vi "Test Child Class Methods.vi"() -> ()   [LabVIEW 2014]
uses:
  TypeDefs/STEP State.ctl
  Measurement/Measurement.lvclass
  STEP/STEP.lvclass
  APIs/Message Queue/Message Cluster.ctl
  AutoZero/AutoZero.lvclass
  Measurement wRelev/Measurement wRelev.lvclass
  Measurement wMaster/Measurement wMaster.lvclass
  Relev/Relev.lvclass
  Mastering/Mastering.lvclass
  Scale Calibration/Scale Calibration.lvclass
  APIs/Message Queue/WINFAS 2 Message Queue.lvlib
  SeqLoop.lvlib
panel:
  out "Array":T1(array[cluster])
  in  "Class":T2(ring)
  in  "STEP State 2":T3=enum."Advance OK"
  in  "STEP State":T3=enum."First Call"
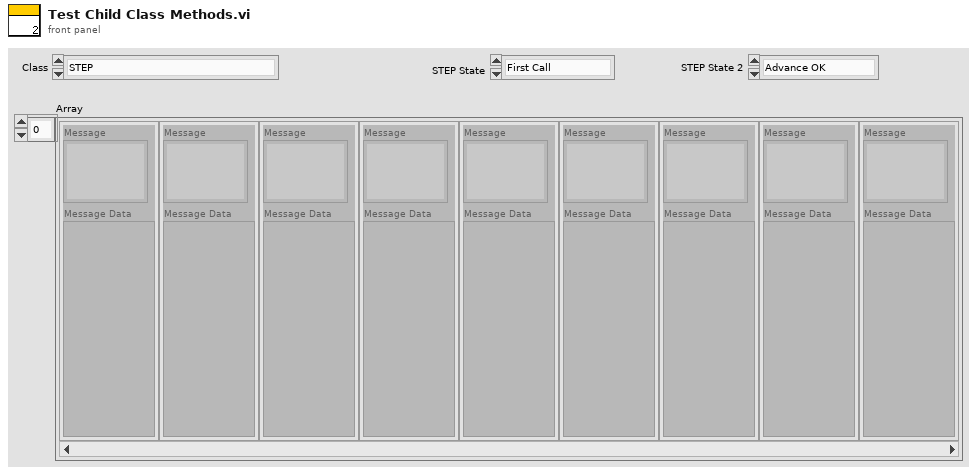
[diagram p1: front panel]
types:
  T1 = cluster{"Message":string, "Message Data":variant}[]
  T2 = enum16{"STEP", "Measurement", "AutoZero", "Measurement wRelev", "Measurement wMaster", "Relev", "Mastering", "Scale Calibration"}
  T3 = typedef "SeqLoop.lvlib/STEP State.ctl" = enum16{"Stopped", "First Call", "Idle...", "Advance OK", "Alarm", "Output Security", "Error"}
  T4 = typedef "WINFAS 2 Message Queue.lvlib/Message Cluster.ctl" = cluster{"Message":string, "Message Data":variant}
  T5 = cluster{"Message":string, "Message Data":variant}
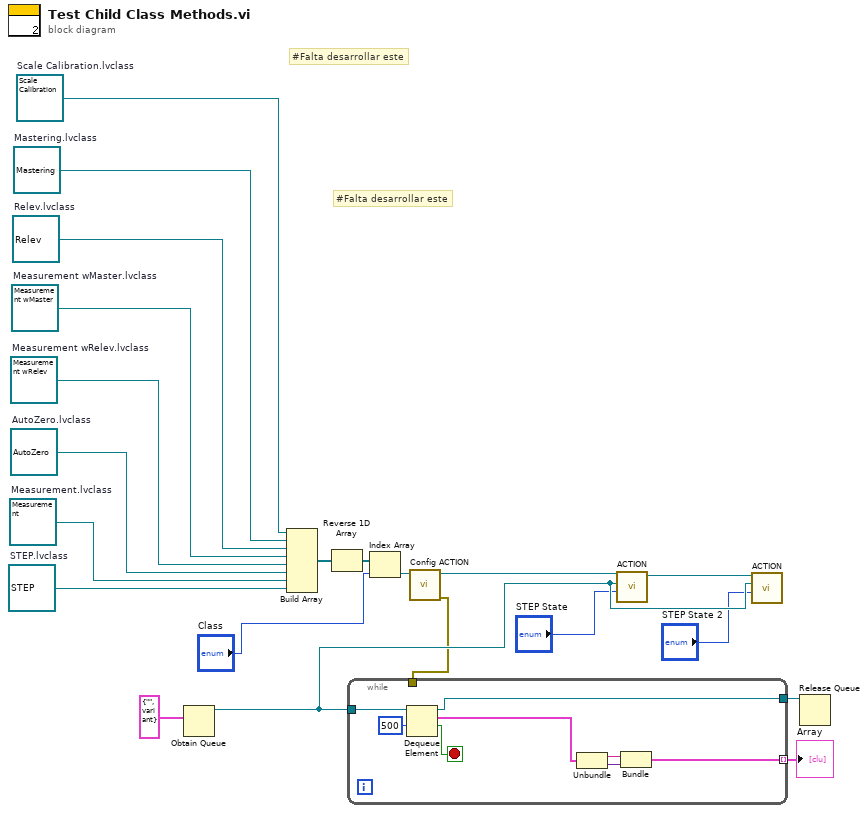
[diagram p0: block diagram]
diagram:
  w5 = refnum<class "Scale Calibration.lvclass"> refnum  # Scale Calibration.lvclass
  w6 = refnum<class "Mastering.lvclass"> refnum  # Mastering.lvclass
  w7 = refnum<class "Relev.lvclass"> refnum  # Relev.lvclass
  w8 = refnum<class "Measurement wMaster.lvclass"> refnum  # Measurement wMaster.lvclass
  w9 = refnum<class "Measurement wRelev.lvclass"> refnum  # Measurement wRelev.lvclass
  w10 = refnum<class "AutoZero.lvclass"> refnum  # AutoZero.lvclass
  w21 = refnum<class "STEP.lvclass"> refnum  # STEP.lvclass
  w17 = refnum<class "Measurement.lvclass"> refnum  # Measurement.lvclass
  # "#Falta desarrollar este"
  # "#Falta desarrollar este"
  n1 = Obtain Queue(element data type=T4 {"Message"="", "Message Data"=variant} ("element")) -> (queue out=w15:refnum<queue>)  [unwired: 4 in, 2 out]
  n2 = Build Array(w5, w6, w7, w8, w9, w10, w17, w21) -> (w3:refnum<class "STEP.lvclass">[])
  n3 = Reverse 1D Array(array=w3) -> (reversed array=w2:refnum<class "STEP.lvclass">[])
  n4 = Index Array(array=w2, index="Class") -> (element=w20:refnum<class "STEP.lvclass">)
  n5 = call-dynamic "Config ACTION.vi"("STEP in"=w20) -> ("error out"=w11:errorcluster, "STEP out"=w19:refnum<class "STEP.lvclass">)  [unwired: 9 in]
  n6 = while {
    tunnel: w15 -> [w29]
    tunnel: [w28] -> w13
    tunnel: w11 -> [_]
    tunnel: [w23] -> w1 mode=indexing
    stop <- w26 stop-if-true
    n7 = Dequeue Element(queue=w29, timeout in ms (-1)=500) -> (queue out=w28:refnum<queue>, element=w25:T4, timed out?=w26:bool)  [unwired: 1 in, 1 out]
    n8 = Unbundle(w25) -> ("Message"=w24:string, "Message Data"=w22:variant)
    n9 = Bundle("Message"=w24, "Message Data"=w22) -> (w23:T5)  [unwired: 1 in]
  }
  "Array" <- w1
  n10 = call-dynamic "ACTION.vi"("STEP State"="STEP State", "CORE"=w15, "STEP in"=w19) -> ("STEP out"=w16:refnum<class "STEP.lvclass">)  [unwired: 7 in, 1 out]
  n11 = call-dynamic "ACTION.vi"("STEP State"="STEP State 2", "CORE"=w15, "STEP in"=w16) -> ()  [unwired: 7 in, 2 out]
  n12 = Release Queue(queue=w13) -> ()  [unwired: 2 in, 3 out]
